vi "Set CDS Loader Ref.vi"(10 "CDS Loader Ref":refnum<vi>, 11 "DMA Channel Testing in":refnum<class "DMA Channel Testing.lvclass">) -> (3 "DMA Channel Testing out":refnum<class "DMA Channel Testing.lvclass">)   [LabVIEW 2019, in "DMA Channel Testing.lvclass"]
uses:
  DMA Channel Testing.lvclass
  DMA Channel Testing.lvclass/DMA Channel Testing.ctl
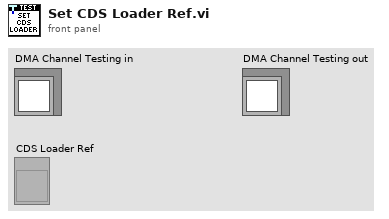
[diagram p1: front panel]
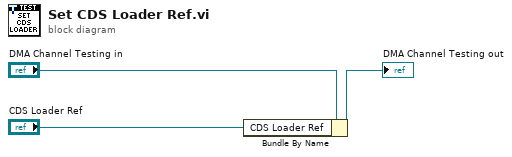
[diagram p0: block diagram]
diagram:
  n1 = Bundle By Name(cluster="DMA Channel Testing in", "CDS Loader Ref"="CDS Loader Ref") -> (→"DMA Channel Testing out":refnum<class "DMA Channel Testing.lvclass">)
